vi "Create All Message Queues.vi"(8 "error in (no error)":errorcluster) -> (0 "error out":errorcluster, 3 "Message Queues out":T1)   [LabVIEW 2014, in "PLS Message Queue.lvlib"]
doc: "This VI creates and initializes all the message queues for your application. If your application requires more than one message queue, right-click the \"Message Queues\" constant above and select Open Type Def. Add the new Message Queue(s) to the type definition, then initialize them in this VI."
uses:
  PLS Message Queue.lvlib
  All Message Queues.ctl
  Message Cluster.ctl
  Enqueue Message (Single).vi
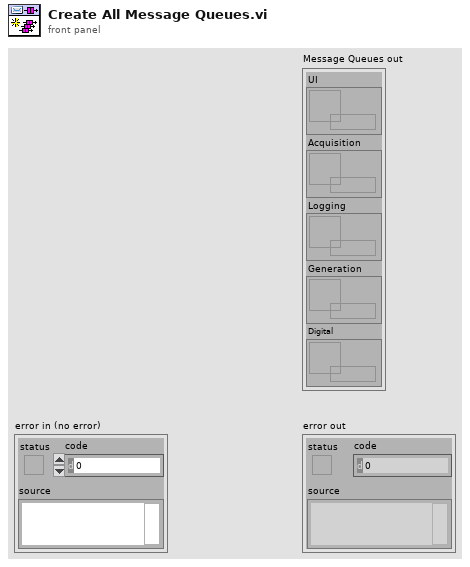
[diagram p1: front panel]
types:
  T1 = typedef "PLS Message Queue.lvlib/All Message Queues.ctl" = cluster{"UI":refnum<queue>, "Acquisition":refnum<queue>, "Logging":refnum<queue>, "Generation":refnum<queue>, "Digital":refnum<queue>}
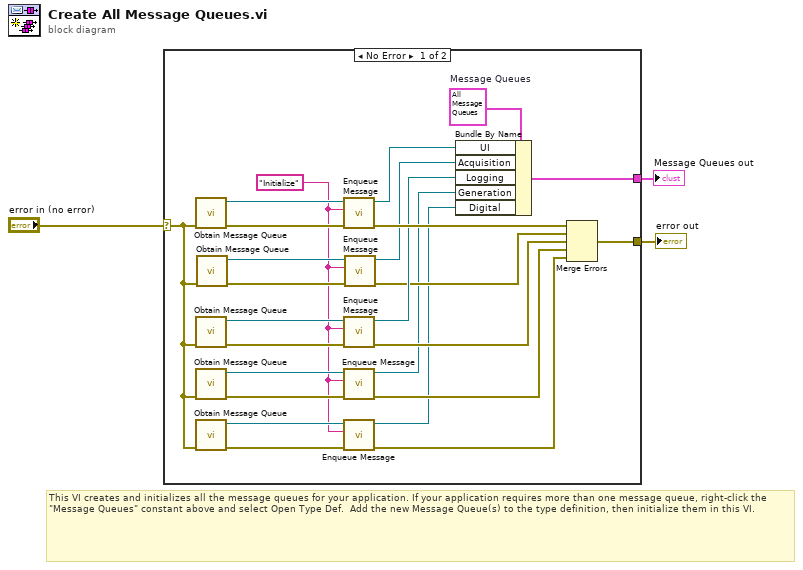
[diagram p0: block diagram]
diagram:
  # "This VI creates and initializes all the message queues for your application. If your application requires more than one message queue, right-click the \"Message Queues\" constant above and select Open Type Def.  Add the new Message Queue(s) to the type definition, then initialize them in this VI."
  n1 = case shown="No Error" "error in (no error)" {
    selector: "error in (no error)" -> [w7 w29]
    tunnel: [w16 w29] -> w3
    tunnel: [w26 _] -> w2
    frame No Error {
      w6 = "Initialize" ("Message")
      w27 = T1 {"UI"=refnum, "Acquisition"=refnum, "Logging"=refnum, "Generation"=refnum, "Digital"=refnum}  # Message Queues
      n2 = call "Obtain Message Queue.vi"("error in (no error)"=w7) -> ("error out"=w25:errorcluster, "Message Queue"=w24:refnum<queue>)  [unwired: 9 in]
      n3 = call "Obtain Message Queue.vi"("error in (no error)"=w7) -> ("error out"=w21:errorcluster, "Message Queue"=w20:refnum<queue>)  [unwired: 9 in]
      n4 = call "Obtain Message Queue.vi"("error in (no error)"=w7) -> ("error out"=w12:errorcluster, "Message Queue"=w13:refnum<queue>)  [unwired: 9 in]
      n5 = call "Obtain Message Queue.vi"("error in (no error)"=w7) -> ("error out"=w9:errorcluster, "Message Queue"=w8:refnum<queue>)  [unwired: 9 in]
      n6 = call "Obtain Message Queue.vi"("error in (no error)"=w7) -> ("error out"=w22:errorcluster, "Message Queue"=w23:refnum<queue>)  [unwired: 9 in]
      n7 = call-poly "Enqueue Message.vi"("error in (no error)"=w25, "Message"=w6, "Message Queue"=w24) -> ("error out"=w28:errorcluster, "dup Message Queue"=w19:refnum<queue>)  [unwired: 7 in]
      n8 = call-poly "Enqueue Message.vi"("error in (no error)"=w21, "Message"=w6, "Message Queue"=w20) -> ("error out"=w14:errorcluster, "dup Message Queue"=w17:refnum<queue>)  [unwired: 7 in]
      n9 = call-poly "Enqueue Message.vi"("error in (no error)"=w12, "Message"=w6, "Message Queue"=w13) -> ("error out"=w11:errorcluster, "dup Message Queue"=w10:refnum<queue>)  [unwired: 7 in]
      n10 = call-poly "Enqueue Message.vi"("error in (no error)"=w9, "Message"=w6, "Message Queue"=w8) -> ("error out"=w4:errorcluster, "dup Message Queue"=w5:refnum<queue>)  [unwired: 7 in]
      n11 = call-poly "Enqueue Message.vi"("error in (no error)"=w22, "Message"=w6, "Message Queue"=w23) -> ("error out"=w15:errorcluster, "dup Message Queue"=w18:refnum<queue>)  [unwired: 7 in]
      n12 = Bundle By Name(cluster=w27, "UI"=w19, "Acquisition"=w18, "Logging"=w17, "Generation"=w10, "Digital"=w5) -> (w26:T1)
      n13 = Merge Errors(w28, w15, w14, w11, w4) -> (w16:errorcluster)
    }
    frame Error {
    }
  }
  "Message Queues out" <- w2
  "error out" <- w3
